vi "LC_Relay_Reclose.vi"(5 "Recloser Settings":T1, 6 "Recloser in":cluster{bool, dbl}, 7 "Reclose?":bool, 8 "VR RMS avg":dbl, 9 "VL RMS avg":dbl, 10 "VR array":waveform(sgl)[](array[waveform]), 11 "VL array":waveform(sgl)[](array[waveform])) -> (0 "Phase difference":dbl, 1 "VR Frequency":dbl, 2 "VL Frequency":dbl, 3 "Recloser action":bool, 4 "Recloser out":cluster{bool, dbl})   [LabVIEW 2016]
doc: "Calculates volatge frequency and angle information.\nChecks voltage magnitude, frequency and angle difference for reclosing."
uses:
  <vilib>/Analysis/3filter.llb/Filter Passband Type.ctl
  <vilib>/Analysis/3filter.llb/Butterworth Filter (DBL).vi
  <vilib>/measure/matone.llb/Extract Single Tone Information N Chan.vi
  <vilib>/measure/NI_MAPro.lvlib
  <vilib>/Analysis/NI_AALBase.lvlib
panel:
  out "frequency difference":dbl
  out "average phase diff":dbl
  out "magnitude difference":dbl
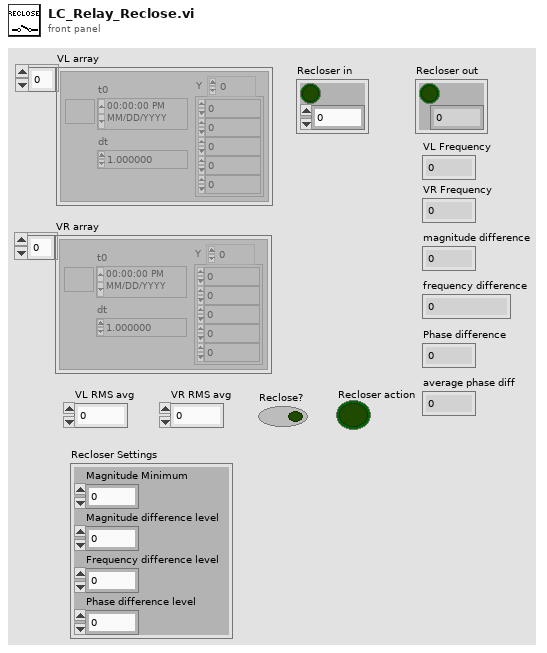
[diagram p1: front panel]
types:
  T1 = cluster{"Magnitude Minimum":dbl, "Magnitude difference level":dbl, "Frequency difference level":dbl, "Phase difference level":dbl}
  T2 = typedef "NI_AALBase.lvlib/Filter Passband Type.ctl" = enum32{"Lowpass", "Highpass", "Bandpass", "Bandstop"}
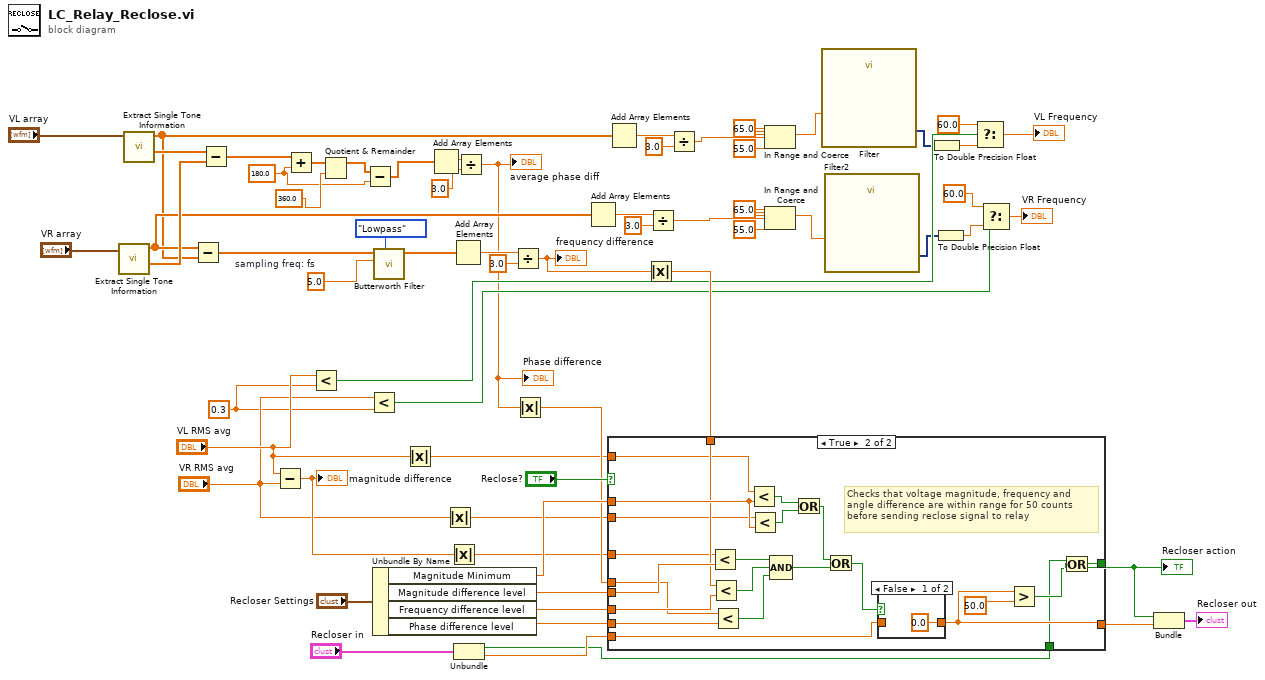
[diagram p0: block diagram]
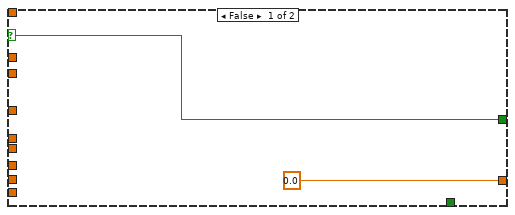
[diagram p2: hidden frame]
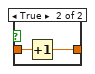
[diagram p3: hidden frame]
diagram:
  w26 = 180.0 ("detected phase (deg)")
  w19 = 0.3 ("y")
  w55 = 5.0  # sampling freq: fs
  n1 = call-poly <vilib>:"Extract Single Tone Information.vi"("time signals in"="VR array") -> ("detected phases (deg)"=w64:dbl[], "detected frequencies"=w38:dbl[])  [unwired: 5 in, 4 out]
  n2 = call-poly <vilib>:"Extract Single Tone Information.vi"("time signals in"="VL array") -> ("detected phases (deg)"=w65:dbl[], "detected frequencies"=w22:dbl[])  [unwired: 5 in, 4 out]
  n3 = Subtract(x=w38, y=w22) -> (x-y=w57:dbl[])
  n4 = Subtract(x=w65, y=w64) -> (x-y=w29:dbl[])
  n5 = Subtract(x="VL RMS avg", y="VR RMS avg") -> (x-y=w49:dbl)
  "magnitude difference" <- w49
  n6 = Add(x=w29, y=w26) -> (x+y=w31:dbl[])
  n7 = Less?(x="VL RMS avg", y=w19) -> (x < y?=w36:bool)
  n8 = Quotient & Remainder(x=w31, y=360.0 ("detected phase (deg)")) -> (x-y*floor(x/y)=w28:dbl[])  [unwired: 1 out]
  n9 = Subtract(x=w28, y=w26) -> (x-y=w27:dbl[])
  n10 = Less?(x="VR RMS avg", y=w19) -> (x < y?=w34:bool)
  n11 = Unbundle By Name("Recloser Settings") -> ("Magnitude Minimum"=w54:dbl, "Magnitude difference level"=w53:dbl, "Frequency difference level"=w52:dbl, "Phase difference level"=w51:dbl)
  n12 = call-poly <vilib>:"Butterworth Filter.vi"("filter type"=Filter_Passband_Type."Lowpass", "sampling freq: fs"=w55, "X"=w57) -> ("Filtered X"=w60:dbl[])  [unwired: 5 in, 1 out]
  n13 = Absolute Value(x="VL RMS avg") -> (abs(x)=w44:dbl)
  n14 = Add Array Elements(numeric array=w27) -> (sum=w62:dbl)
  n15 = Absolute Value(x="VR RMS avg") -> (abs(x)=w45:dbl)
  n16 = Absolute Value(x=w49) -> (abs(x)=w46:dbl)
  n17 = Add Array Elements(numeric array=w60) -> (sum=w59:dbl)
  n18 = Unbundle("Recloser in") -> (w13:bool, w14:dbl)
  n19 = Divide(x=w62, y=3.0 ("x")) -> (x/y=w20:dbl)
  "average phase diff" <- w20
  "Phase difference" <- w20
  n20 = Divide(x=w59, y=3.0) -> (x/y=w50:dbl)
  "frequency difference" <- w50
  n21 = Absolute Value(x=w20) -> (abs(x)=w47:dbl)
  n22 = Add Array Elements(numeric array=w38) -> (sum=w40:dbl)
  n23 = Add Array Elements(numeric array=w22) -> (sum=w23:dbl)
  n24 = Absolute Value(x=w50) -> (abs(x)=w43:dbl)
  n25 = case shown="True" "Reclose?" {
    selector: "Reclose?" -> [w67 _]
    tunnel: [w67 w68] -> w18
    tunnel: [0.0 w70] -> w17
    tunnel: w54 -> [_ w82]
    tunnel: w53 -> [_ w81]
    tunnel: w52 -> [_ w80]
    tunnel: w51 -> [_ w79]
    tunnel: w47 -> [_ w78]
    tunnel: w43 -> [_ w77]
    tunnel: w46 -> [_ w76]
    tunnel: w14 -> [_ w75]
    tunnel: w44 -> [_ w74]
    tunnel: w45 -> [_ w73]
    tunnel: w13 -> [_ w69]
    frame False {
    }
    frame True {
      # "Checks that voltage magnitude, frequency and \nangle difference are within range for 50 counts\nbefore sending reclose signal to relay"
      n26 = Less?(x=w76, y=w81) -> (x < y?=w85:bool)
      n27 = Less?(x=w77, y=w80) -> (x < y?=w88:bool)
      n28 = Less?(x=w78, y=w79) -> (x < y?=w87:bool)
      n29 = Less?(x=w74, y=w82) -> (x < y?=w90:bool)
      n30 = Less?(x=w73, y=w82) -> (x < y?=w89:bool)
      n31 = Compound Arithmetic op=AND(w85, w88, w87) -> (w86:bool)
      n32 = Or(x=w90, y=w89) -> (x .or. y?=w84:bool)
      n33 = Or(x=w84, y=w86) -> (x .or. y?=w83:bool)
      n34 = case shown="False" w83 {
        tunnel: [0.0 w93] -> w70
        tunnel: w75 -> [_ w92]
        frame False {
        }
        frame True {
          n35 = Increment(x=w92) -> (x+1=w93:dbl)
        }
      }
      n36 = Greater?(x=w70, y=50.0 ("x")) -> (0:w72:bool)
      n37 = Or(x=w69, y=w72) -> (x .or. y?=w68:bool)
    }
  }
  "Recloser action" <- w18
  n38 = Divide(x=w40, y=3.0) -> (x/y=w1:dbl)
  n39 = Divide(x=w23, y=3.0) -> (x/y=w5:dbl)
  n40 = In Range and Coerce(upper limit=65.0, x=w5, lower limit=55.0) -> (coerced(x)=w6:dbl)  [unwired: 1 out]
  n41 = In Range and Coerce(upper limit=65.0, x=w1, lower limit=55.0) -> (coerced(x)=w2:dbl)  [unwired: 1 out]
  n42 = call "Filter"("Signal"=w6) -> ("Filtered Signal"=w11:dynamicdata)  [unwired: 9 in, 1 out]
  n43 = call "Filter2"("Signal"=w2) -> ("Filtered Signal"=w9:dynamicdata)  [unwired: 9 in, 1 out]
  n44 = To Double Precision Float(number=w11) -> (double precision float=w12:dbl)
  n45 = To Double Precision Float(number=w9) -> (double precision float=w10:dbl)
  n46 = Select(t=60.0, s=w36, f=w12) -> (s? t:f=→"VL Frequency":dbl)
  n47 = Select(t=60.0, s=w34, f=w10) -> (s? t:f=→"VR Frequency":dbl)
  n48 = Bundle(w18, w17) -> (→"Recloser out":cluster{bool, dbl})  [unwired: 1 in]
